vi "Create Frame.vi"(6 "Type":T1, 7 "Input?":bool, 8 "error in (no error)":errorcluster, 10 "Frame":T3 {"Signals"."Byte Order" items=["Little Endian", "Big Endian"]; "Signals"."Data Type" items=["Signed", "Unsigned", "IEEE Float"]}, 11 "Section Ptr":T2 format="%.0x") -> (0 "error out":errorcluster, 3 "Parent Ref out":T2 format="%.0x")   [LabVIEW 2015, in "Diagnostics Addon System Explorer.lvlib"]
uses:
  System Explorer/Diagnostics Addon System Explorer.lvlib
  Frame Parameters.ctl
  Signal Parameters.ctl
  <vilib>/NI Veristand/Custom Device API/Custom Device Item Ref.ctl
  System Explorer/SubVIs/Frame Type.ctl
  FG Action.ctl
  <vilib>/NI Veristand/Custom Device API/NI VeriStand - Get Item Property.vi
  <vilib>/NI Veristand/Custom Device API/Get Item Property (U32).vi
  <vilib>/NI Veristand/Custom Device API/NI VeriStand - Set Item Property.vi
  <vilib>/NI Veristand/Custom Device API/Set Item Property (U32).vi
  GUID Lookup.vi
  <vilib>/NI Veristand/Custom Device API/Custom Device API.lvlib
  Diagnostics Addon Shared.lvlib
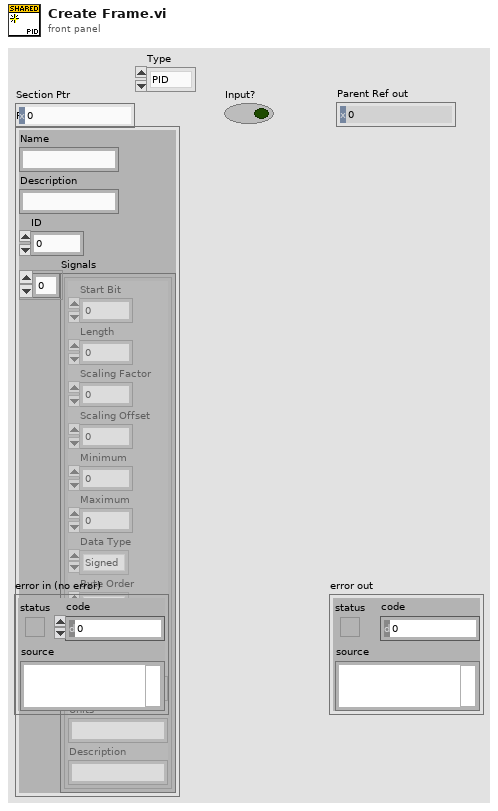
[diagram p1: front panel]
types:
  T1 = typedef "Diagnostics Addon System Explorer.lvlib/Frame Type.ctl" = enum8{"PID", "DID", "Memory"}
  T2 = typedef "Custom Device API.lvlib/Custom Device Item Ref.ctl" = u64
  T3 = typedef "Diagnostics Addon Shared.lvlib/Frame Parameters.ctl" = cluster{"Name":string, "Description":string, "ID":u16, "Signals":T4[]}
  T4 = typedef "Diagnostics Addon Shared.lvlib/Signal Parameters.ctl" = cluster{"Start Bit":u8, "Length":u8, "Scaling Factor":dbl, "Scaling Offset":dbl, "Minimum":dbl, "Maximum":dbl, "Data Type":u32, "Byte Order":u32, "Default Value":dbl, "Name":string, "Units":string, "Description":string}
  T5 = typedef "Diagnostics Addon System Explorer.lvlib/FG Action.ctl" = enum16{"Get", "Set"}
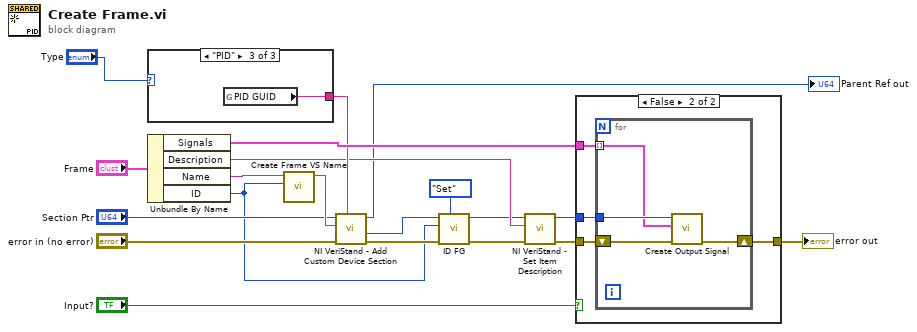
[diagram p0: block diagram]
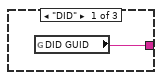
[diagram p2: hidden frame]
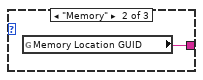
[diagram p3: hidden frame]
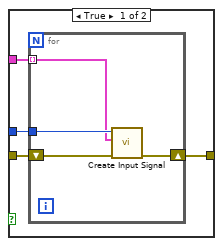
[diagram p4: hidden frame]
diagram:
  n1 = case shown="\"PID\"" "Type" {
    tunnel: [w21 w22 w23] -> w15
    frame "DID" {
      n2 = global read "GUID Lookup.vi" "DID GUID"() -> (w21:string)
    }
    frame "Memory" {
      n3 = global read "GUID Lookup.vi" "Memory Location GUID"() -> (w22:string)
    }
    frame "PID" {
      n4 = global read "GUID Lookup.vi" "PID GUID"() -> (w23:string)
    }
  }
  n5 = Unbundle By Name("Frame") -> ("Signals"=w18:T4[], "Description"=w9:string, "Name"=w19:string, "ID"=w2:u16)
  n6 = call "Create Frame VS Name.vi"("PID Number"=w2, "PID Name"=w19) -> ("VS Name"=w20:string)  [unwired: 9 in]
  n7 = call <vilib>:"NI VeriStand - Add Custom Device Section.vi"("GUID (Default Section)"=w15, "error in (no error)"="error in (no error)", "Section Name"=w20, "Parent Ref in"="Section Ptr") -> ("error out"=w6:errorcluster, "Section Ptr"=w4:T2, "Parent Ref out"=→"Parent Ref out":T2)  [unwired: 4 in, 1 out]
  n8 = call "ID FG.vi"("Action"=FG_Action."Set", "error in (no error)"=w6, "ID"=w2, "Device Item Ref in"=w4) -> ("error out"=w5:errorcluster, "Device Item Ref out"=w3:T2)  [unwired: 5 in, 1 out]
  n9 = call <vilib>:"NI VeriStand - Set Item Description.vi"("error in (no error)"=w5, "Description"=w9, "Item Ref in"=w3) -> ("error out"=w13:errorcluster, "Item Ref out"=w12:T2)  [unwired: 6 in, 1 out]
  n10 = case shown="False" "Input?" {
    tunnel: w12 -> [w27 w35]
    tunnel: w18 -> [w26 w34]
    tunnel: [w25 w33] -> w17
    tunnel: w13 -> [w24 w32]
    frame True {
      n11 = for {
        shift-right: [w30] -> w25
        shift-left: w24 -> [w31]
        tunnel: w26 -> [w28] mode=indexing
        tunnel: w27 -> [w29]
        n12 = call "Create Input Signal.vi"("error in (no error)"=w31, "Signal Parameters"=w28, "Section Ptr"=w29) -> ("error out"=w30:errorcluster)  [unwired: 7 in, 1 out]
      }
    }
    frame False {
      n13 = for {
        shift-right: [w36] -> w33
        shift-left: w32 -> [w38]
        tunnel: w34 -> [w37] mode=indexing
        tunnel: w35 -> [w39]
        n14 = call "Create Output Signal.vi"("error in (no error)"=w38, "Signal Parameters"=w37, "Section Ptr"=w39) -> ("error out"=w36:errorcluster)  [unwired: 7 in, 1 out]
      }
    }
  }
  "error out" <- w17
